vi "txt reader.vi"(4 "data info template":refnum<vi>, 5 "duration of zero (index)":i32=1000, 6 "ADC ZERO drifts are taken into account !":bool, 7 "start zero index":i32=100, 8 "error in (no error)":errorcluster, 9 "sampling rate, Hz":dbl[](array[numeric]) format="%.2f", 10 "file paths":path[](array[path]), 11 "how many files":i32) -> (0 "error out":errorcluster, 1 "source txt":T1, 2 "channels quantity in file":i32[](array[numeric]), 3 "ActiveChannelsArray":i32[][](array[numeric]))   [LabVIEW 2014]
uses:
  <vilib>/Analysis/baseanly.llb/Mean (DBL).vi
  <vilib>/Utility/file.llb/Read From Spreadsheet File (DBL).vi
  <vilib>/Waveform/WDTOps.llb/WDT Get Waveform Subset DBL.vi
  <vilib>/Analysis/NI_AALBase.lvlib
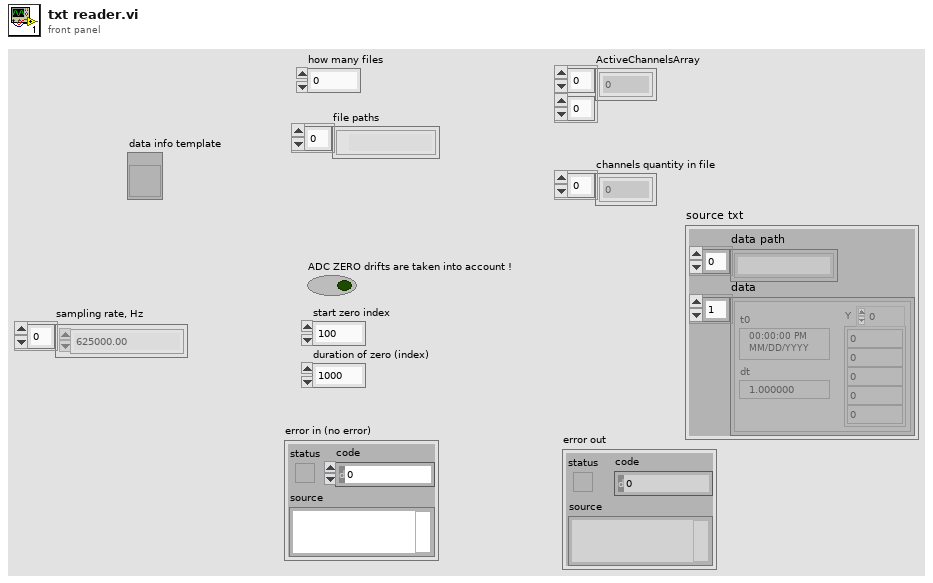
[diagram p1: front panel]
types:
  T1 = cluster{"data path":string[], "data":waveform(dbl)[]}
  T2 = cluster{"data path":string, "ADCintercadr_s":dbl, "data info":cluster{"use or not *.info.txt?":i16, "probe name":string, "signal type":string, "Unit":string, "variable":string, "attenuation factor":dbl, "amplification factor":dbl, "extracoef#1":dbl, "extracoef#2":dbl, "U cascade, kV":string, "probe area, cm2":dbl, "plasma, a.m.u.":dbl}, "channel_name":string, "channels_in_file":i32, "LastModified":string}
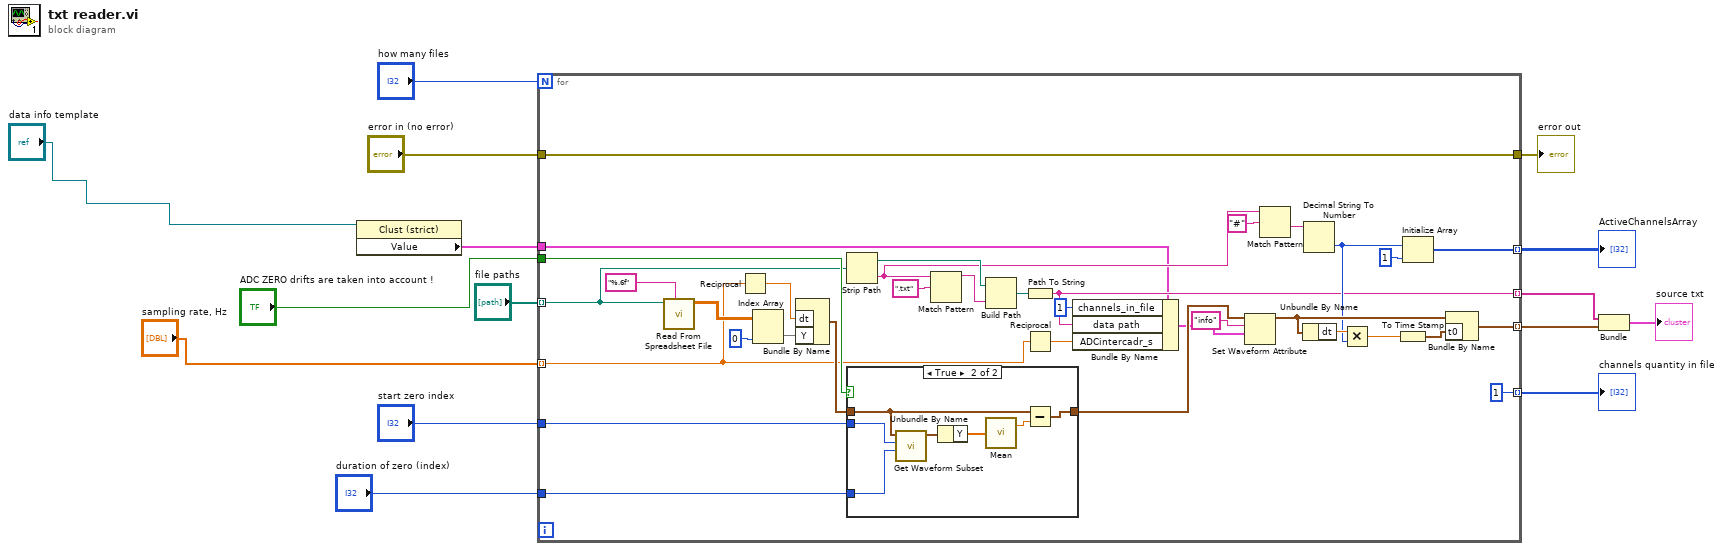
[diagram p0: block diagram]
diagram:
  n1 = property on="Property Node" class="Clust (strict)"(reference="data info template") -> ("Value"=w4:T2)  [unwired: 1 in, 2 out]
  n2 = for {
    N: "how many files" -> [_]
    tunnel: "file paths" -> [w24] mode=indexing
    tunnel: [w38] -> w3 mode=indexing
    tunnel: [1] -> w14 mode=indexing
    tunnel: [w48] -> w13 mode=indexing
    tunnel: [w25] -> w12
    tunnel: "ADC ZERO drifts are taken into account !" -> [w45]
    tunnel: "start zero index" -> [w44]
    tunnel: "duration of zero (index)" -> [w43]
    tunnel: "error in (no error)" -> [w25]
    tunnel: [w33] -> w6 mode=indexing
    tunnel: w4 -> [w18]
    tunnel: "sampling rate, Hz" -> [w16] mode=indexing
    n3 = call-poly <vilib>:"Read From Spreadsheet File.vi"("format (%.3f)"="%.6f", "file path (dialog if empty)"=w24) -> ("all rows"=w30:dbl[][])  [unwired: 5 in, 4 out]
    n4 = Reciprocal(x=w16) -> (1/x=w27:dbl)
    n5 = Index Array(array=w30, index (col)=0 ("dimension size")) -> (element=w28:dbl[])  [unwired: 1 in]
    n6 = Bundle By Name("dt"=w27, "Y"=w28) -> (w26:waveform(dbl))  [unwired: 1 in]
    n7 = Strip Path(path=w24) -> (stripped path=w23:path, name=w22:string)
    n8 = case shown="True" w45 {
      tunnel: w44 -> [_ w53]
      tunnel: w43 -> [_ w52]
      tunnel: [w51 w55] -> w46
      tunnel: w26 -> [w51 w54]
      frame False {
      }
      frame True {
        n9 = call-poly <vilib>:"Get Waveform Subset.vi"("duration"=w52, "start samples/time"=w53, "waveform in"=w54) -> ("waveform out"=w57:waveform(dbl))  [unwired: 3 in, 3 out]
        n10 = Unbundle By Name(w57) -> ("Y"=w58:dbl[])
        n11 = call-poly <vilib>:"Mean.vi"("X"=w58) -> ("mean"=w56:dbl)  [unwired: 1 out]
        n12 = Subtract(x=w54, y=w56) -> (x-y=w55:waveform(dbl))
      }
    }
    n13 = Match Pattern(string=w22, regular expression=".txt") -> (before substring=w20:string)  [unwired: 1 in, 3 out]
    n14 = Build Path(base path=w23, name or relative path=w20) -> (appended path=w19:path)
    n15 = Path To String(path=w19) -> (string=w33:string)
    n16 = Reciprocal(x=w16) -> (1/x=w37:dbl)
    n17 = Bundle By Name(cluster=w18, "channels_in_file"=1, "data path"=w33, "ADCintercadr_s"=w37) -> (w32:T2)
    n18 = Set Waveform Attribute(5:w32, 6:"info" ("name"), 7:w46) -> (3:w39:waveform(dbl))  [unwired: 1 in, 2 out]
    n19 = Match Pattern(string=w22, regular expression="#") -> (after substring=w35:string)  [unwired: 1 in, 3 out]
    n20 = Unbundle By Name(w39) -> ("dt"=w41:dbl)
    n21 = Decimal String To Number(string=w35) -> (number=w34:i32)  [unwired: 2 in, 1 out]
    n22 = Multiply(x=w41, y=w34) -> (x*y=w40:dbl)
    n23 = To Time Stamp(1:w40) -> (0:w42:timestamp)
    n24 = Initialize Array(w34, 1 ("dimension size")) -> (w48:i32[])
    n25 = Bundle By Name(cluster=w39, "t0"=w42) -> (w38:waveform(dbl))
  }
  "channels quantity in file" <- w14
  "ActiveChannelsArray" <- w13
  "error out" <- w12
  n26 = Bundle "Bundle"(w6, w3) -> (→"source txt":cluster{string[], waveform(dbl)[]})  [unwired: 1 in]
